vi "Property Node_Colors and Icons.vi"(11 "Property Type":T2(ring)=enum."Base") -> (1 "Icon Pixmap":T1, 2 "Icon Picture":picture, 3 "Color":u32(colorbox)=16777164)   [LabVIEW 2023]
doc: "Return the background colors for the four types of property nodes. Examples of the nodes are on the block diagram.\n\nAlso returns a 16x16 icon that can be used in a tree control."
panel:
  # "See block diagram"
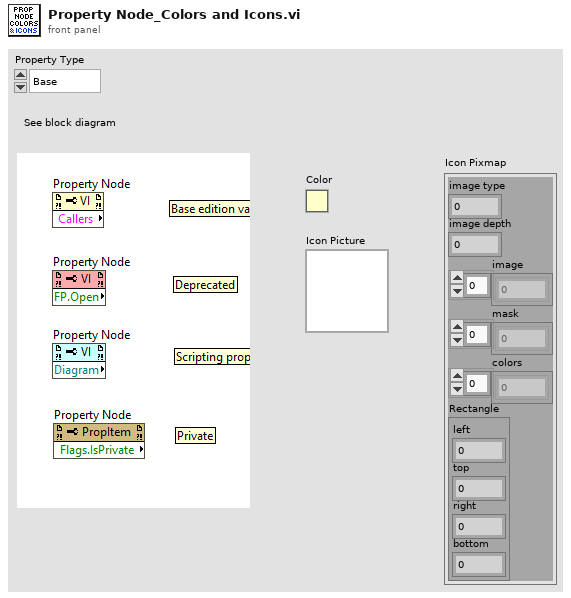
[diagram p1: front panel]
types:
  T1 = cluster{"image type":i32, "image depth":i32, "image":u8[], "mask":u8[], "colors":u32[], "Rectangle":cluster{"left":i16, "top":i16, "right":i16, "bottom":i16}}
  T2 = enum16{"Unknown", "Base", "Scripting", "Private", "Deprecated", "None", "Divider"}
  T3 = typedef "imagedata.ctl" = cluster{"image type":i32, "image depth":i32, "image":u8[], "mask":u8[], "colors":u32[], "Rectangle":cluster{"left":i16, "top":i16, "right":i16, "bottom":i16}}
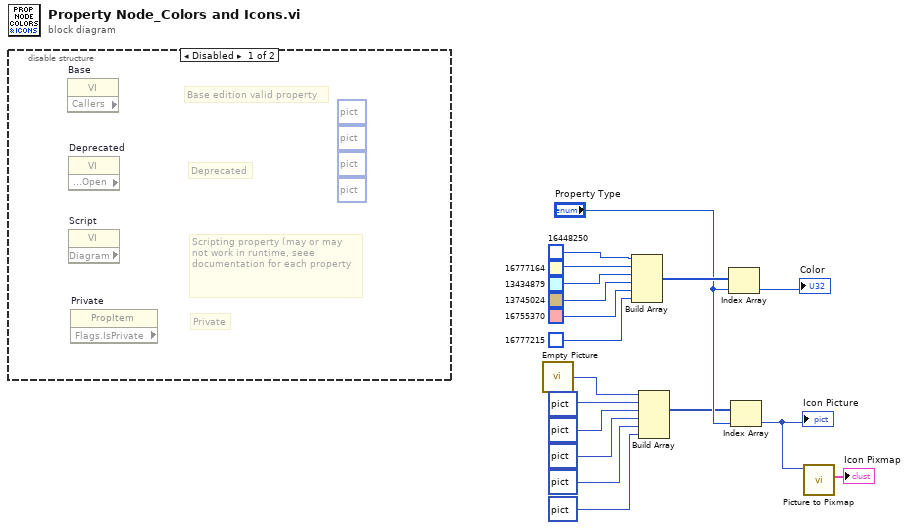
[diagram p0: block diagram]
diagram:
  n1 = disable-structure shown="Disabled" {
    frame Disabled {
      w20 = picture bytes[2374] ("Scripting")
      w19 = picture bytes[2374] ("Base")
      w22 = picture bytes[2374] ("Deprecated")
      w21 = picture bytes[2374] ("Private")
      # "Private"
      # "Scripting property (may or may not work in runtime, seee documentation for each property"
      # "Base edition valid property"
      # "Deprecated"
      n2 = property on="Base" class="VI" props=["Callers"]() -> ()  [unwired: 2 in, 3 out]
      n3 = property on="Deprecated" class="VI" props=["Front Panel.Open"]() -> ()  [unwired: 2 in, 3 out]
      n4 = property on="Script" class="VI" props=["Diagram"]() -> ()  [unwired: 2 in, 3 out]
      n5 = property on="Private" class="PropItem" props=["Flags.IsPrivate"]() -> ()  [unwired: 2 in, 3 out]
    }
    frame Enabled {
    }
  }
  n6 = call "Empty Picture"() -> ("empty picture"=w4:picture)
  n7 = Build Array(u32 16448250 ("Color"), u32 16777164 ("Color"), u32 13434879 ("Scripting Color"), u32 13745024 ("Private Color"), u32 16755370 ("Deprecated Color"), u32 16777215 ("Deprecated Color")) -> (w14:u32[])
  n8 = Build Array(w4, picture bytes[2294] ("Private"), picture bytes[2294] ("Deprecated"), picture bytes[2294] ("Base"), picture bytes[2294] ("Scripting"), picture bytes[580] ("Scripting")) -> (w7:picture[])
  n9 = Index Array(array=w14, index="Property Type") -> (element=→"Color":u32)
  n10 = Index Array(array=w7, index="Property Type") -> (element=w6:picture)
  "Icon Picture" <- w6
  n11 = call <vilib>:"Picture to Pixmap.vi"("picture"=w6) -> ("image data"=→"Icon Pixmap":T3)  [unwired: 9 in, 1 out]
